vi "setIndex.vi"(10 "Index":i32, 11 "ModbusBuffer in":refnum<class "ModbusBufferBuilder.lvclass">) -> (3 "ModbusBuffer out":refnum<class "ModbusBufferBuilder.lvclass">)   [LabVIEW 2016, in "ModbusBufferBuilder.lvclass"]
uses:
  ModbusBufferBuilder.lvclass
  ModbusBufferBuilder.lvclass/ModbusBufferBuilder.ctl
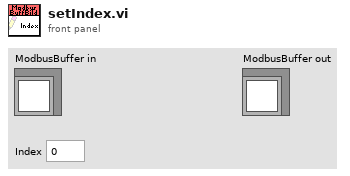
[diagram p1: front panel]
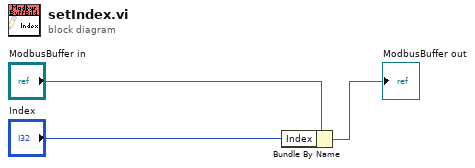
[diagram p0: block diagram]
diagram:
  n1 = Bundle By Name(cluster="ModbusBuffer in", "Index"="Index") -> (→"ModbusBuffer out":refnum<class "ModbusBufferBuilder.lvclass">)
